vi "Initialize Analog Data Array.vi"(8 "error in":errorcluster, 11 "AnalogInput in":refnum<class "AnalogInput.lvclass">) -> (0 "error out":errorcluster, 3 "AnalogInput out":refnum<class "AnalogInput.lvclass">)   [LabVIEW 2019, in "AnalogInput.lvlib" / "AnalogInput.lvclass"]
doc: "This vi should only be called after the information regarding the number of channels has been loaded from the configuration file."
uses:
  Library/AnalogInput.lvclass
  Library/AnalogInput.lvclass/AnalogInput.ctl
  Custom Controls/Range.ctl
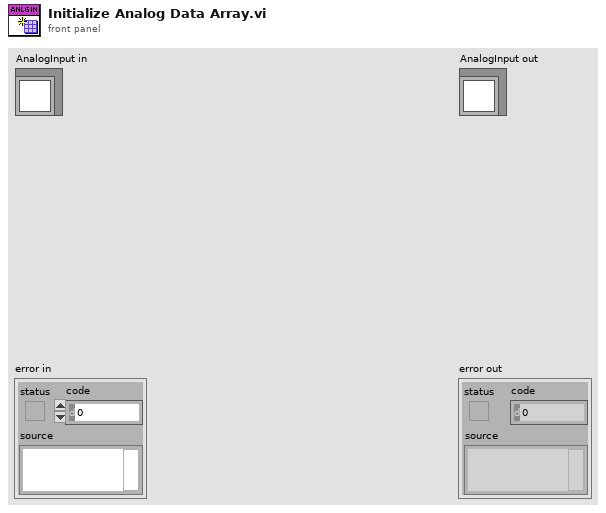
[diagram p1: front panel]
types:
  T1 = typedef "AnalogInput.lvlib/AnalogInput.lvclass/Range.ctl" = cluster{"Max Value":dbl, "Min Value":dbl}
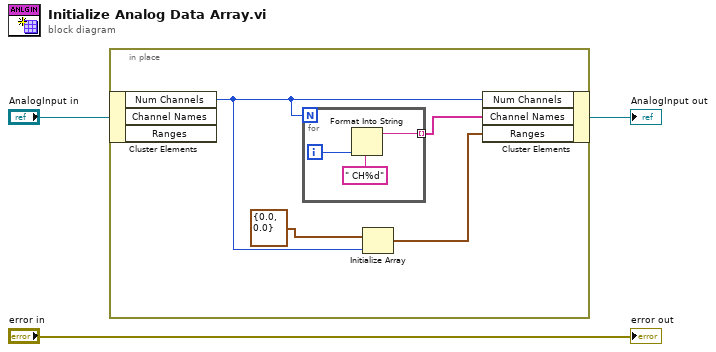
[diagram p0: block diagram]
diagram:
  n1 = in-place {
    n2 = in-place-cluster #1("AnalogInput in") -> ("Num Channels"=w5:u32)  [unwired: 2 out]
    n3 = for {
      N: w5 -> [_]
      tunnel: [w8] -> w4 mode=indexing
      i -> [w10]
      n4 = Format Into String(format string=" CH%d", w10) -> (resulting string=w8:string)  [unwired: 2 in, 1 out]
    }
    n5 = Initialize Array(T1 {"Max Value"=0.0, "Min Value"=0.0} ("Range"), w5) -> (w6:T1[])
    n6 = in-place-cluster #1("Num Channels"=w5, "Channel Names"=w4, "Ranges"=w6) -> (→"AnalogInput out":refnum<class "AnalogInput.lvclass">)
  }
  "error out" <- "error in"
